vi "swap cloumns.vi"(9 "columns":string[](array[string]), 10 "表格":string[][](table), 11 "交换参数":cluster{"移动前":i32, "移动后":i32}[](array[cluster])) -> (2 "columns 2":string[](array[string]), 3 "表格 2":string[][](array[string]))   [LabVIEW 2016]
panel:
  in  "数据表":T1
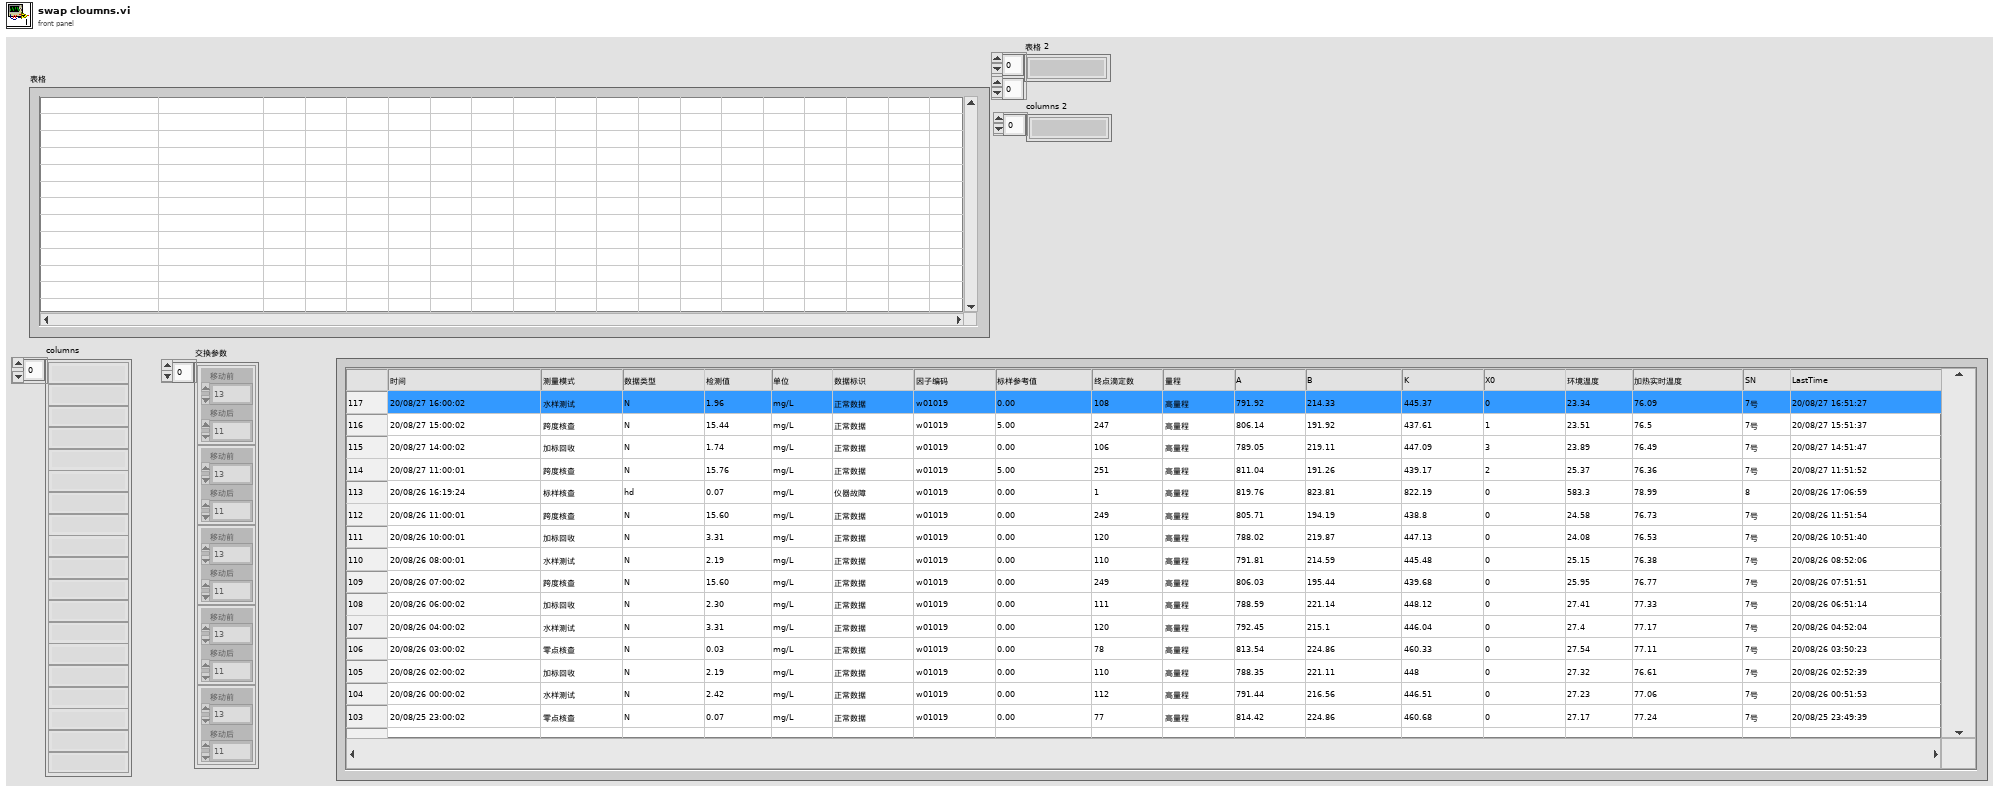
[diagram p1: front panel]
types:
  T1 = typedef "数据查询大列表框.ctl" = i32
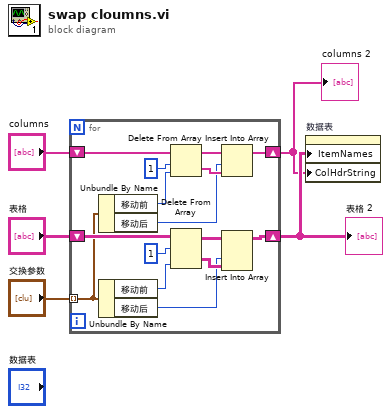
[diagram p0: block diagram]
diagram:
  n1 = for {
    tunnel: "交换参数" -> [w10] mode=indexing
    shift-right: [w14] -> w2
    shift-left: "表格" -> [w17]
    shift-right: [w6] -> w1
    shift-left: "columns" -> [w11]
    n2 = Unbundle By Name(w10) -> ("移动前"=w9:i32, "移动后"=w7:i32)
    n3 = Unbundle By Name(w10) -> ("移动前"=w16:i32, "移动后"=w15:i32)
    n4 = Delete From Array(array=w11, length=1 ("长度"), index=w9) -> (deleted portion=w8:string[], array with subset deleted=w12:string[])
    n5 = Delete From Array(array=w17, length=1 ("长度"), index (col)=w16) -> (deleted portion=w19:string[][], array with subset deleted=w20:string[][])  [unwired: 1 in]
    n6 = Insert Into Array(array=w12, index=w7, new element=w8) -> (w6:string[])
    n7 = Insert Into Array(array=w20, index (col)=w15, new element=w19) -> (w14:string[][])  [unwired: 1 in]
  }
  "表格 2" <- w2
  "columns 2" <- w1
  n8 = property on="数据表" class="MCListbox (严格)"("ItemNames"=w2, "ColHdrString"=w1) -> ()  [unwired: 2 in, 2 out]
